vi "ExternalCBTemplate.vi"(8 "error in (no error)":errorcluster, 11 "Message to LabVIEW App":T1={"Command"="zxcvbnm,", "Data"=["asdfghjk", "qwertyui"], "Script ID"=0, "LabVIEW Server ID"="localhost:9007", "Python Message ID"=0}) -> (0 "error out":errorcluster)   [LabVIEW 2013, in "TS.lvlib"]
doc: "Use this template to send a message to your LabVIEW app, using whatever communication means you like - queues, notifiers, actors, etc."
uses:
  TS.lvlib
  LabVIEW Python Connector Message.ctl
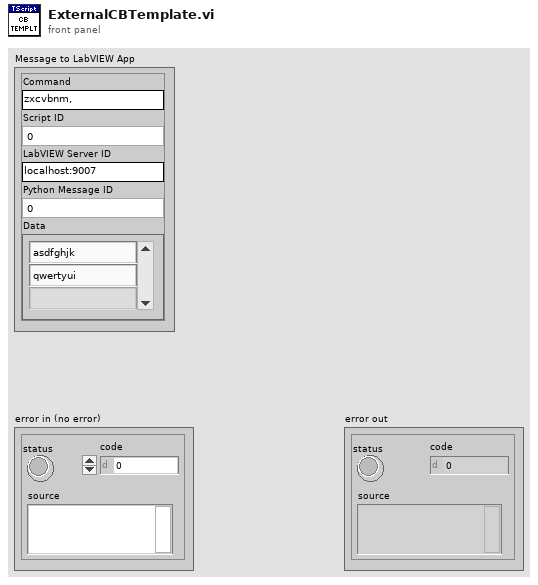
[diagram p1: front panel]
types:
  T1 = typedef "TS.lvlib/LabVIEW Python Connector Message.ctl" = cluster{"Command":string, "Data":string[], "Script ID":i64, "LabVIEW Server ID":string, "Python Message ID":i32}
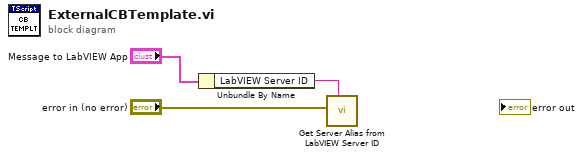
[diagram p0: block diagram]
diagram:
  n1 = Unbundle By Name("Message to LabVIEW App") -> ("LabVIEW Server ID"=w1:string)
  n2 = call "Get Server Alias from LabVIEW Server ID.vi"("LabVIEW Server ID"=w1, "Error In"="error in (no error)") -> ()  [unwired: 8 in, 2 out]
